vi "Player Info.vi"(11 "Starter In":refnum<class "Starter.lvclass">) -> (0 "Defeat Speech":string, 1 "Victory Speech":string, 2 "Name":string, 3 "Starter Out":refnum<class "Starter.lvclass">)   [LabVIEW 2015, in "Starter.lvclass"]
uses:
  Starter.lvclass
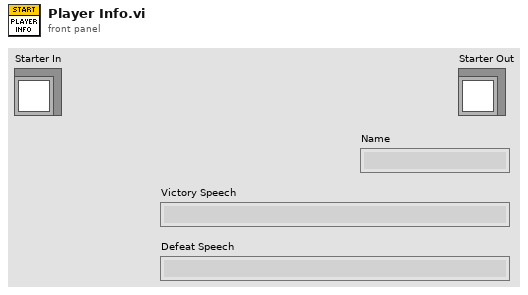
[diagram p1: front panel]
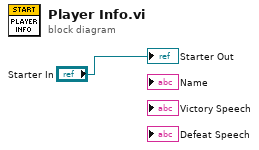
[diagram p0: block diagram]
diagram:
  "Starter Out" <- "Starter In"
